vi "Read Byte.vi"(7 "1-Wire DIO Pin":refnum<k21>="ConnectorA/DIO15", 8 "error in":errorcluster) -> (0 "error out":errorcluster, 2 "Bit Array":bool[](array[boolean]))   [LabVIEW 2014, in "Maxim 1-Wire.lvlib"]
doc: "This VI is created by Vincent Claes for FPDA-1 more information on http://pwo.fpga.be\n\nvincent.claes@xios.be\nclaesvincent@gmail.com\n\nhttp://www.linkedin.com/in/vincentclaes"
uses:
  Maxim 1-Wire.lvlib
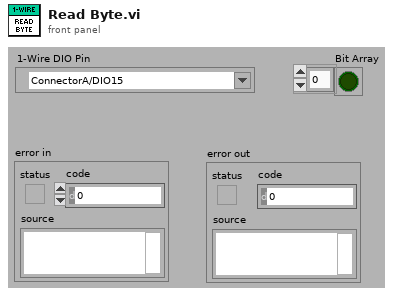
[diagram p1: front panel]
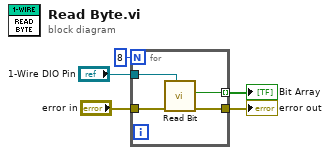
[diagram p0: block diagram]
diagram:
  n1 = for {
    N: 8 -> [_]
    tunnel: [w9] -> w5 mode=indexing
    tunnel: "error in" -> [w8]
    tunnel: [w7] -> w2
    tunnel: "1-Wire DIO Pin" -> [w6]
    n2 = call "Read Bit.vi"("1-Wire DIO Pin"=w6, "error in"=w8) -> ("error out"=w7:errorcluster, "Bit Read"=w9:bool)  [unwired: 8 in]
  }
  "Bit Array" <- w5
  "error out" <- w2
